vi "CalcDeltaPhase.vi"(5 "CrossNew":bool, 7 "CoNew":bool, 10 "Cross":T1 {"Beac"."Tone"."median" format="%0.2f"; "Beac"."Tone"."MaxQ" format="%0.2f"; "Cal"."Tone"."median" format="%0.2f"; "Cal"."Tone"."MaxQ" format="%0.2f"}, 11 "Co":T1 {"Beac"."Tone"."median" format="%0.2f"; "Beac"."Tone"."MaxQ" format="%0.2f"; "Cal"."Tone"."median" format="%0.2f"; "Cal"."Tone"."MaxQ" format="%0.2f"}) -> (3 "output cluster":T1={"Cal"={"Shift_"=-24999462.633451957, "Peak_ToFPGA"=-24999462.633451957, "MaxValue"=0.0, "MaxIndex"=0, "Tone"={"PkLocTrak"=0.0, "PkLocDisp"=0.0, "df_"=0.0, "ZoomPwr"=[], "Phase"=0.0, "PhaseOld"=0.0, "AboveThresh?"=FALSE, "MaxI"=0.0, "MaxQ"=0.0, "median"=0.0, "ISpect"=[], "QSpect"=[], "DeltaPhase"=0.0}, "TimeDomainI"=array[12500 elements], "TimeDomainQ"=array[12500 elements], "PwrSpectrum"=[], "RunningAvgFreq"=0.0, "ISpectPos"=[], "ISpectNeg"=[], "QSpectPos"=[], "QSpectNeg"=[], "10Hz_PwrSpectr"=[], "SNR"=0.0, "AliasWarn"=FALSE, "10Hz_Peak"=[], "ISpect+-"=[], "QSpect+-"=[], "TimeStamp"=timestamp(0 s since 1904-01-01), "I_Index"=array[12500 elements], "Q_Index"=array[12500 elements], "10MHz"=FALSE}, "Beac"={"Shift_"=-24999462.633451957, "Peak_ToFPGA"=-24999462.633451957, "MaxValue"=0.0, "MaxIndex"=0, "Tone"={"PkLocTrak"=0.0, "PkLocDisp"=0.0, "df_"=0.0, "ZoomPwr"=[], "Phase"=0.0, "PhaseOld"=0.0, "AboveThresh?"=FALSE, "MaxI"=0.0, "MaxQ"=0.0, "median"=0.0, "ISpect"=[], "QSpect"=[], "DeltaPhase"=0.0}, "TimeDomainI"=array[12500 elements], "TimeDomainQ"=array[12500 elements], "PwrSpectrum"=[], "RunningAvgFreq"=0.0, "ISpectPos"=[], "ISpectNeg"=[], "QSpectPos"=[], "QSpectNeg"=[], "10Hz_PwrSpectr"=[], "SNR"=0.0, "AliasWarn"=FALSE, "10Hz_Peak"=[], "ISpect+-"=[], "QSpect+-"=[], "TimeStamp"=timestamp(0 s since 1904-01-01), "I_Index"=array[12500 elements], "Q_Index"=array[12500 elements], "10MHz"=FALSE}, "Time"=[], "Saturat"={"MeasMean0"=0.0, "MeasMean1"=0.0, "MeasMax"=0.0, "1_Max"=0.0, "4_Max"=0.0, "5_Max"=0.0, "6_Max"=0.0, "7_Max"=0.0}} {"Beac"."Tone"."median" format="%0.2f"; "Beac"."Tone"."MaxQ" format="%0.2f"; "Cal"."Tone"."median" format="%0.2f"; "Cal"."Tone"."MaxQ" format="%0.2f"})   [LabVIEW 2018]
uses:
  Controls/Clusts/TargetToneData.ctl
  Controls/Clusts/ChannelToneData.ctl
  Controls/ToneInfoClust.ctl
  Controls/Clusts/SaturationMonitor.ctl
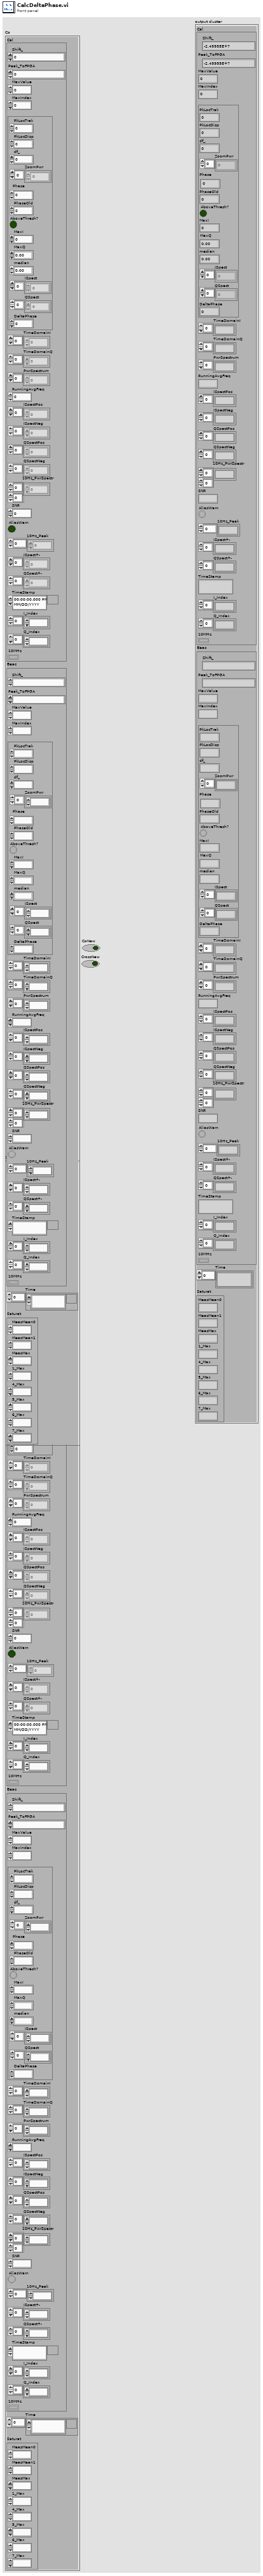
[diagram p1: front panel]
types:
  T1 = typedef "TargetToneData.ctl" = cluster{"Cal":T2, "Beac":T2, "Time":timestamp[], "Saturat":T4}
  T2 = typedef "ChannelToneData.ctl" = cluster{"Shift_":dbl, "Peak_ToFPGA":dbl, "MaxValue":dbl, "MaxIndex":i32, "Tone":T3, "TimeDomainI":ext[], "TimeDomainQ":ext[], "PwrSpectrum":dbl[], "RunningAvgFreq":dbl, "ISpectPos":dbl[], "ISpectNeg":dbl[], "QSpectPos":dbl[], "QSpectNeg":dbl[], "10Hz_PwrSpectr":dbl[][], "SNR":dbl, "AliasWarn":bool, "10Hz_Peak":dbl[], "ISpect+-":dbl[], "QSpect+-":dbl[], "TimeStamp":timestamp, "I_Index":ext[], "Q_Index":ext[], "10MHz":bool}
  T3 = typedef "ToneInfoClust.ctl" = cluster{"PkLocTrak":dbl, "PkLocDisp":dbl, "df_":dbl, "ZoomPwr":dbl[], "Phase":dbl, "PhaseOld":dbl, "AboveThresh?":bool, "MaxI":dbl, "MaxQ":dbl, "median":dbl, "ISpect":dbl[], "QSpect":dbl[], "DeltaPhase":dbl}
  T4 = typedef "SaturationMonitor.ctl" = cluster{"MeasMean0":dbl, "MeasMean1":dbl, "MeasMax":dbl, "1_Max":dbl, "4_Max":dbl, "5_Max":dbl, "6_Max":dbl, "7_Max":dbl}
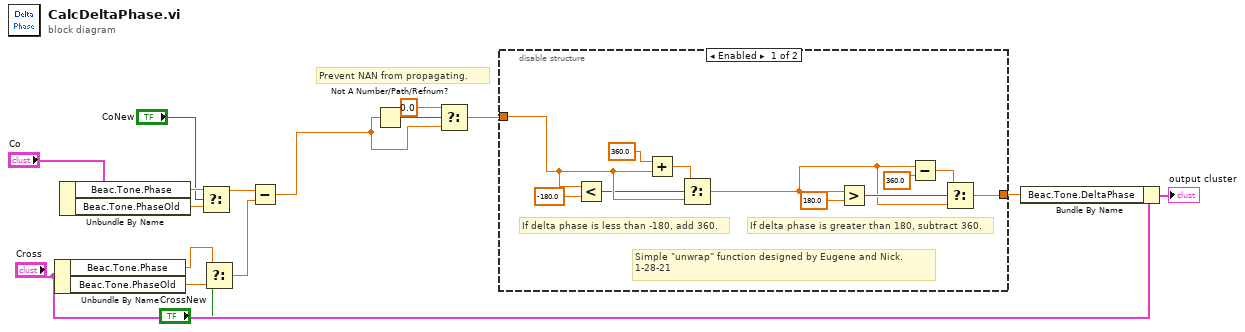
[diagram p0: block diagram]
diagram:
  # "Prevent NAN from propagating."
  n1 = Unbundle By Name("Cross") -> ("Beac.Tone.Phase"=w3:dbl, "Beac.Tone.PhaseOld"=w2:dbl)
  n2 = Unbundle By Name("Co") -> ("Beac.Tone.Phase"=w16:dbl, "Beac.Tone.PhaseOld"=w6:dbl)
  n3 = Select(t=w16, s="CoNew", f=w6) -> (s? t:f=w7:dbl)
  n4 = Select(t=w3, s="CrossNew", f=w2) -> (s? t:f=w4:dbl)
  n5 = Subtract(x=w7, y=w4) -> (x-y=w10:dbl)
  n6 = Not A Number/Path/Refnum?(number/path/refnum=w10) -> (NaN/Path/Refnum?=w12:bool)
  n7 = Select(t=0.0 ("element"), s=w12, f=w10) -> (s? t:f=w9:dbl)
  n8 = disable-structure shown="Enabled" {
    disable-tunnel: w9 -> [w27 w28]
    disable-tunnel: [w19 w28] -> w8
    frame Enabled {
      # "Simple \"unwrap\" function designed by Eugene and Nick.\n1-28-21"
      # "If delta phase is greater than 180, subtract 360."
      # "If delta phase is less than -180, add 360."
      n9 = Less?(x=w27, y=-180.0 ("x")) -> (x < y?=w25:bool)
      n10 = Add(x=360.0 ("y"), y=w27) -> (x+y=w26:dbl)
      n11 = Select(t=w26, s=w25, f=w27) -> (s? t:f=w20:dbl)
      n12 = Greater?(x=w20, y=180.0 ("x")) -> (0:w22:bool)
      n13 = Subtract(x=w20, y=360.0) -> (x-y=w21:dbl)
      n14 = Select(t=w21, s=w22, f=w20) -> (s? t:f=w19:dbl)
    }
    frame Disabled {
    }
  }
  n15 = Bundle By Name(cluster="Cross", "Beac.Tone.DeltaPhase"=w8) -> (→"output cluster":T1)
